vi "VI Tree.vi"   [LabVIEW 2024, in "Bronkhorst FLOW-BUS.lvlib"]
doc: "This is the instrument driver for Bronkhorst FLOW-BUS Instruments. The VI Tree displays all the user-callable VIs of the instrument driver in an organized table."
uses:
  Bronkhorst FLOW-BUS.lvlib
  Configure/Setpoint/Configure Setpoint (Direct).vi
  Data/Setpoint/Read Setpoint (Direct).vi
  Data/Measure/Read Measure (Percentage).vi
panel:
  # "(c) 2014 Bronkhorts High-Tech B.V.  ALL RIGHTS RESERVED."
  # "SEE DIAGRAM\nFOR VI TREE."
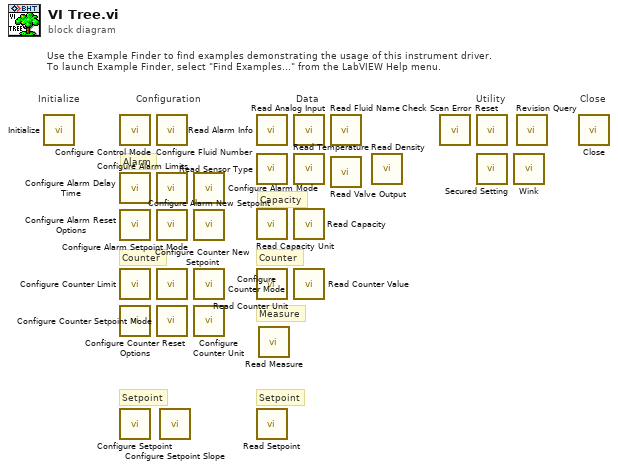
[diagram p0: block diagram]
diagram:
  # "Setpoint"
  # "Counter"
  # "Measure"
  # "Setpoint"
  # "Counter"
  # "Capacity"
  # "Alarm"
  # "Use the Example Finder to find examples demonstrating the usage of this instrument driver.\nTo launch Example Finder, select \"Find Examples...\" from the LabVIEW Help menu."
  # "Configuration"
  # "Utility"
  # "Data"
  # "Close"
  # "Initialize"
  n1 = call "Initialize.vi"() -> ()  [unwired: 10 in, 2 out]
  n2 = call "Configure Control Mode.vi"() -> ()  [unwired: 10 in, 2 out]
  n3 = call "Configure Alarm Delay Time.vi"() -> ()  [unwired: 10 in, 2 out]
  n4 = call "Configure Alarm Reset Options.vi"() -> ()  [unwired: 10 in, 2 out]
  n5 = call "Configure Counter Limit.vi"() -> ()  [unwired: 10 in, 2 out]
  n6 = call "Configure Counter Reset Options.vi"() -> ()  [unwired: 10 in, 2 out]
  n7 = call-poly "Configure Setpoint.vi"() -> ()  [unwired: 10 in, 2 out]
  n8 = call "Configure Fluid Number.vi"() -> ()  [unwired: 10 in, 2 out]
  n9 = call "Configure Alarm Limits.vi"() -> ()  [unwired: 10 in, 2 out]
  n10 = call "Configure Alarm Setpoint Mode.vi"() -> ()  [unwired: 10 in, 2 out]
  n11 = call "Configure Counter New Setpoint.vi"() -> ()  [unwired: 10 in, 2 out]
  n12 = call "Configure Counter Setpoint Mode.vi"() -> ()  [unwired: 10 in, 2 out]
  n13 = call "Configure Setpoint Slope.vi"() -> ()  [unwired: 10 in, 2 out]
  n14 = call "Configure Alarm Mode.vi"() -> ()  [unwired: 10 in, 2 out]
  n15 = call "Configure Alarm New Setpoint.vi"() -> ()  [unwired: 10 in, 2 out]
  n16 = call "Configure Counter Mode.vi"() -> ()  [unwired: 10 in, 2 out]
  n17 = call "Configure Counter Unit.vi"() -> ()  [unwired: 10 in, 2 out]
  n18 = call "Read Alarm Info.vi"() -> ()  [unwired: 9 in, 3 out]
  n19 = call "Read Sensor Type.vi"() -> ()  [unwired: 8 in, 4 out]
  n20 = call "Read Capacity Unit.vi"() -> ()  [unwired: 9 in, 3 out]
  n21 = call "Read Counter Unit.vi"() -> ()  [unwired: 9 in, 3 out]
  n22 = call-poly "Read Setpoint.vi"() -> ()  [unwired: 9 in, 3 out]
  n23 = call-poly "Read Measure.vi"() -> ()  [unwired: 9 in, 3 out]
  n24 = call "Read Analog Input.vi"() -> ()  [unwired: 9 in, 3 out]
  n25 = call "Read Temperature.vi"() -> ()  [unwired: 9 in, 3 out]
  n26 = call "Read Capacity.vi"() -> ()  [unwired: 9 in, 3 out]
  n27 = call "Read Counter Value.vi"() -> ()  [unwired: 9 in, 3 out]
  n28 = call "Read Fluid Name.vi"() -> ()  [unwired: 9 in, 3 out]
  n29 = call "Read Valve Output.vi"() -> ()  [unwired: 8 in, 4 out]
  n30 = call "Read Density.vi"() -> ()  [unwired: 9 in, 3 out]
  n31 = call "Check Scan Error.vi"() -> ()  [unwired: 9 in, 3 out]
  n32 = call "Reset.vi"() -> ()  [unwired: 10 in, 2 out]
  n33 = call "Secured Setting.vi"() -> ()  [unwired: 10 in, 2 out]
  n34 = call "Wink.vi"() -> ()  [unwired: 10 in, 2 out]
  n35 = call "Revision Query.vi"() -> ()  [unwired: 7 in, 5 out]
  n36 = call "Close.vi"() -> ()  [unwired: 11 in, 1 out]
